vi "RestoreWindow.vi"(8 "No Error":errorcluster, 11 "Window [SDL_Window *]":T1 format="%.0x") -> (0 "Error Out":errorcluster)   [LabVIEW 2026, in "SDL3.lvlib" / "Video.lvlib"]
doc: "<B>Summary</B>\nRequest that the size and position of a minimized or maximized window be restored.\n\n<B>Remarks</B>\nOn some windowing systems this request is asynchronous and the new window state may not have have been applied immediately upon the return of this function. If an immediate change is required, call <B>SDL_SyncWindow()</B> to block until the changes have taken effect.\n\nWhen the window state changes, an <B>SDL_EVENT_WINDOW_RESTORED</B> event will be emitted. Note that, as this is just a request, the windowing system can deny the state change."
uses:
  Video.lvlib
  <vilib>/Utility/error.llb/Error Cluster From Error Code.vi
  Error/Error.lvlib
  Lib/SDL3.dll
  SDL_Window--pointer.ctl
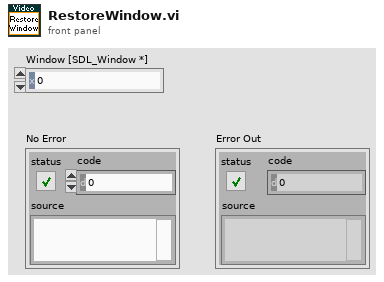
[diagram p1: front panel]
types:
  T1 = typedef "SDL3.lvlib/Video.lvlib/SDL_Window--pointer.ctl" = i64
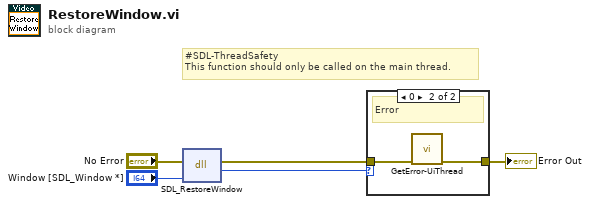
[diagram p0: block diagram]
diagram:
  # "#SDL-ThreadSafety\nThis function should only be called on the main thread."
  n1 = dll-call lib="C:/Users/saukko/Dev/LV-SDL3/Sources/SDL3/Lib/SDL3.*" fn="SDL_RestoreWindow"(error in="No Error", "window"="Window [SDL_Window *]") -> (error out=w3:errorcluster, "return type"=w1:i32)  [unwired: 3 in, 1 out]
  n2 = case shown="0" w1 {
    tunnel: w3 -> [w6 w8]
    tunnel: [w6 w7] -> w2
    frame Default {
      # "Ok"
    }
    frame 0 {
      # "Error"
      n3 = call "GetError-UiThread.vi"("No Error"=w8) -> ("error out"=w7:errorcluster)  [unwired: 10 in]
    }
  }
  "Error Out" <- w2
